vi "Add Data Sharing Framework with UDP Component.vi"(10 "Input System Definition File":path=path "../Assets/Empty.nivssdf", 11 "Output System Definition File":path=path "../Assets/DSF_UDP_Loopback.nivssdf") -> (3 "Created System Definition File":path)   [LabVIEW 2020, in "Data Sharing Framework Scripting Examples.lvlib"]
doc: "Demonstrates using the Data Sharing Framework scripting API to add a UDP plugin for data communication."
uses:
  Data Sharing Framework Scripting Examples.lvlib
  <vilib>/addons/VeriStand Custom Device Scripting APIs/Data Sharing Framework/DSF Core.lvlibp/Typedefs/DSF Engine Framework Configuration.ctl
  <vilib>/addons/VeriStand Custom Device Scripting APIs/Data Sharing Framework/DSF Core.lvlibp/Typedefs/DSF Engine Plugin Configuration.ctl
  <vilib>/addons/VeriStand Custom Device Scripting APIs/Data Sharing Framework/DSF Core.lvlibp/Typedefs/Core Plugin Configuration.ctl
  <vilib>/addons/VeriStand Custom Device Scripting APIs/Data Sharing Framework/DSF Core.lvlibp/Typedefs/DSF Timing Info.ctl
  <vilib>/addons/VeriStand Custom Device Scripting APIs/Data Sharing Framework/DSF Core.lvlibp/Typedefs/DSF Settings Info.ctl
  <vilib>/addons/VeriStand Custom Device Scripting APIs/Data Sharing Framework/DSF Core.lvlibp/Typedefs/DSF Engine Plugin Thread Configuration.ctl
  <vilib>/addons/VeriStand Custom Device Scripting APIs/Data Sharing Framework/DSF Core.lvlibp/Typedefs/Core Thread Configuration.ctl
  <vilib>/addons/VeriStand Custom Device Scripting APIs/Data Sharing Framework/DSF Core.lvlibp/Typedefs/DSF Engine Transfer Group Configuration.ctl
  <vilib>/addons/VeriStand Custom Device Scripting APIs/Data Sharing Framework/DSF Core.lvlibp/Typedefs/Core Group Configuration.ctl
  <vilib>/addons/VeriStand Custom Device Scripting APIs/Data Sharing Framework/DSF Core.lvlibp/Typedefs/DSF Direction.ctl
  <vilib>/addons/VeriStand Custom Device Scripting APIs/Data Sharing Framework/DSF Core.lvlibp/Typedefs/DSF Timeout Behavior.ctl
  <vilib>/addons/VeriStand Custom Device Scripting APIs/Data Sharing Framework/DSF Core.lvlibp/Typedefs/DSF Engine Transfer Configuration.ctl
  <vilib>/addons/VeriStand Custom Device Scripting APIs/Data Sharing Framework/DSF Core.lvlibp/Typedefs/Core Transfer Configuration.ctl
  <vilib>/addons/VeriStand Custom Device Scripting APIs/Data Sharing Framework/DSF Core.lvlibp/Typedefs/DSF Engine Channel Configuration.ctl
  <vilib>/addons/VeriStand Custom Device Scripting APIs/Data Sharing Framework/DSF Core.lvlibp/Typedefs/Core Channel Configuration.ctl
  <vilib>/addons/VeriStand Custom Device Scripting APIs/Data Sharing Framework/DSF Core.lvlibp/Typedefs/DSF Data Type.ctl
  NationalInstruments.VeriStand.SystemDefinitionAPI
  <vilib>/addons/VeriStand Custom Device Scripting APIs/Data Sharing Framework/DSF Core.lvlibp
  <vilib>/addons/VeriStand Custom Device Scripting APIs/Data Sharing Framework/DSF Core.lvlibp/Classes/Configuration/Core/Channel/Channel Configuration.lvclass
  <vilib>/addons/VeriStand Custom Device Scripting APIs/Data Sharing Framework/DSF Core.lvlibp/Classes/Configuration/Core/Transfer/Transfer Configuration.lvclass
  <vilib>/addons/VeriStand Custom Device Scripting APIs/Data Sharing Framework/DSF Core.lvlibp/Classes/Configuration/Core/Group/Group Configuration.lvclass
  <vilib>/addons/VeriStand Custom Device Scripting APIs/Data Sharing Framework/DSF Core.lvlibp/Classes/Configuration/Core/Thread/Thread Configuration.lvclass
  <vilib>/addons/VeriStand Custom Device Scripting APIs/Data Sharing Framework/DSF Core.lvlibp/Classes/Configuration/Core/Plugin/Plugin Configuration.lvclass
  <vilib>/addons/VeriStand Custom Device Scripting APIs/Data Sharing Framework/Data Sharing Framework Custom Device Scripting.lvlib
panel:
  in  "Launch Data Viewer":bool=TRUE
  in  "Data Server Frequency":dbl(ring)=10.0 items=["0.5 Hz"=0.5, "1.0 Hz"=1.0, "2.0 Hz"=2.0, "2.5 Hz"=2.5, "4.0 Hz"=4.0, "5.0 Hz"=5.0, "8.0 Hz"=8.0, "10.0 Hz"=10.0, "12.5 Hz"=12.5, "20.0 Hz"=20.0, "25.0 Hz"=25.0, "40.0 Hz"=40.0, "50.0 Hz"=50.0, "100.0 Hz"=100.0]
  in  "Enable Data Server":bool=TRUE
  in  "Channels":cluster{"Name":string, "Unit":string}[](array[cluster])=[{"Name"="Voltage_an", "Unit"="V"}, {"Name"="Voltage_bn", "Unit"="V"}, {"Name"="Voltage_cn", "Unit"="V"}, {"Name"="Current_a", "Unit"="A"}, {"Name"="Current_b", "Unit"="A"}, {"Name"="Current_c", "Unit"="A"}, {"Name"="Current_n", "Unit"="A"}, {"Name"="Voltage_dc", "Unit"="V"}, {"Name"="Current_dc", "Unit"="A"}, {"Name"="Count", "Unit"="iterations"}]
  # "Overview: Demonstrates using the Data Sharing Framework scripting API to add a UDP plugin for data communication. \n\nInstructions:\n1. Per your application requirements, configure the data channels to share.\n2. Browse to a path to save the system definition file as the output Output System Definition File.  This may be the same as the input file.\n3. Run the VI and verify the resulting system definition file. \n4. Configure addresses and ports in System Explorer."
  # "System Definition Files"
  # "Configure Data Server for Validation"
  # "Data Sharing Framework Channels"
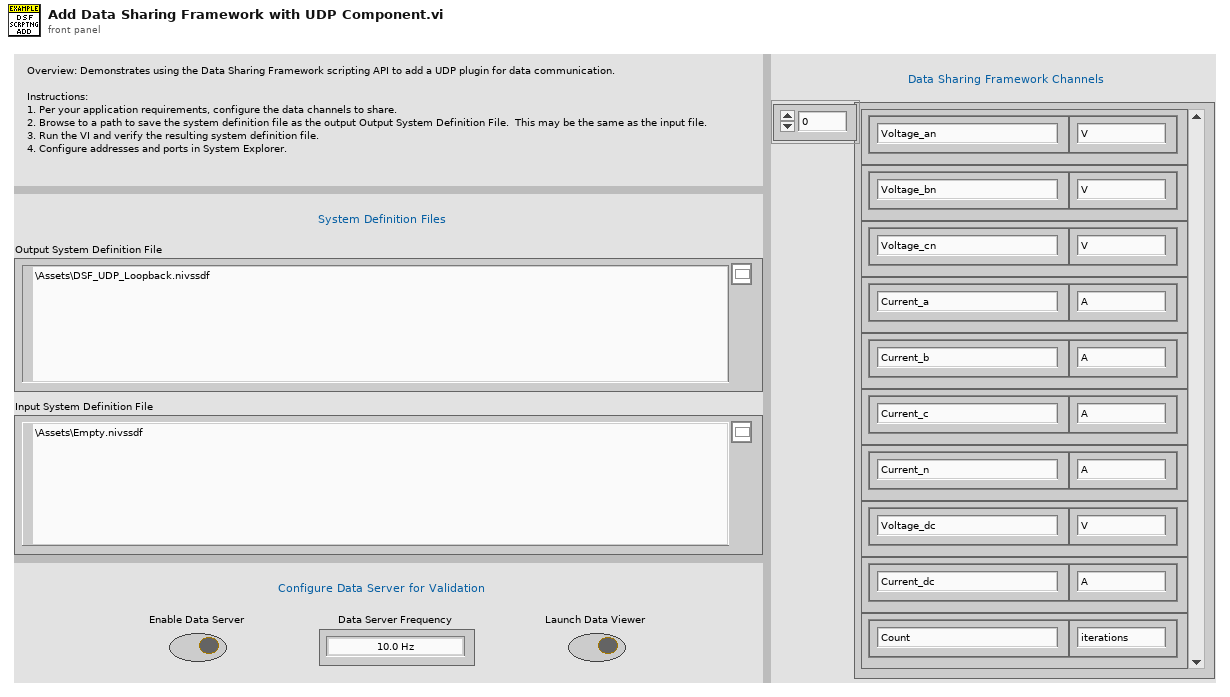
[diagram p1: front panel]
types:
  T1 = typedef "DSF Core.lvlibp/DSF Engine Channel Configuration.ctl" = cluster{"core":T2, "component settings":T4[]}
  T2 = typedef "DSF Core.lvlibp/Channel Configuration.lvclass/Core Channel Configuration.ctl" = cluster{"name":string, "units":string, "engine data type":T3, "string data type":T3, "string offset":u64}
  T3 = typedef "DSF Core.lvlibp/DSF Data Type.ctl" = enum8{"Bool", "SGL", "DBL", "I8", "I16", "I32", "I64", "U8", "U16", "U32", "U64"}
  T4 = typedef "DSF Core.lvlibp/DSF Settings Info.ctl" = cluster{"component":string, "values":cluster{"key":string, "value":string}[]}
  T5 = typedef "DSF Core.lvlibp/DSF Engine Plugin Thread Configuration.ctl" = cluster{"core":T6, "component settings":T4[], "transfer groups":T7[]}
  T6 = typedef "DSF Core.lvlibp/Thread Configuration.lvclass/Core Thread Configuration.ctl" = cluster{"processor":i32, "priority offset":i16}
  T7 = typedef "DSF Core.lvlibp/DSF Engine Transfer Group Configuration.ctl" = cluster{"core":T8, "component settings":T4[], "transfers":T12[]}
  T8 = typedef "DSF Core.lvlibp/Group Configuration.lvclass/Core Group Configuration.ctl" = cluster{"name":string, "direction":T9, "cycle timing":T10, "timeout behavior":T11, "enable conversion":bool}
  T9 = typedef "DSF Core.lvlibp/DSF Direction.ctl" = enum8{"Tx", "Rx"}
  T10 = typedef "DSF Core.lvlibp/DSF Timing Info.ctl" = cluster{"priority":u64, "decimation":u64, "offset":u64}
  T11 = typedef "DSF Core.lvlibp/DSF Timeout Behavior.ctl" = enum8{"Increment Late Count", "Throw Error"}
  T12 = typedef "DSF Core.lvlibp/DSF Engine Transfer Configuration.ctl" = cluster{"core":T13, "component settings":T4[], "channels":T1[]}
  T13 = typedef "DSF Core.lvlibp/Transfer Configuration.lvclass/Core Transfer Configuration.ctl" = cluster{"name":string}
  T14 = typedef "DSF Core.lvlibp/DSF Engine Plugin Configuration.ctl" = cluster{"core":T15, "component settings":T4[], "threads":T5[]}
  T15 = typedef "DSF Core.lvlibp/Plugin Configuration.lvclass/Core Plugin Configuration.ctl" = cluster{"name":string, "components":string[], "cycle timing":T10}
  T16 = typedef "DSF Core.lvlibp/DSF Engine Framework Configuration.ctl" = cluster{"plugins":T14[]}
  T17 = typedef "Custom Device API.lvlib/Custom Device Item Ref.ctl" = u64
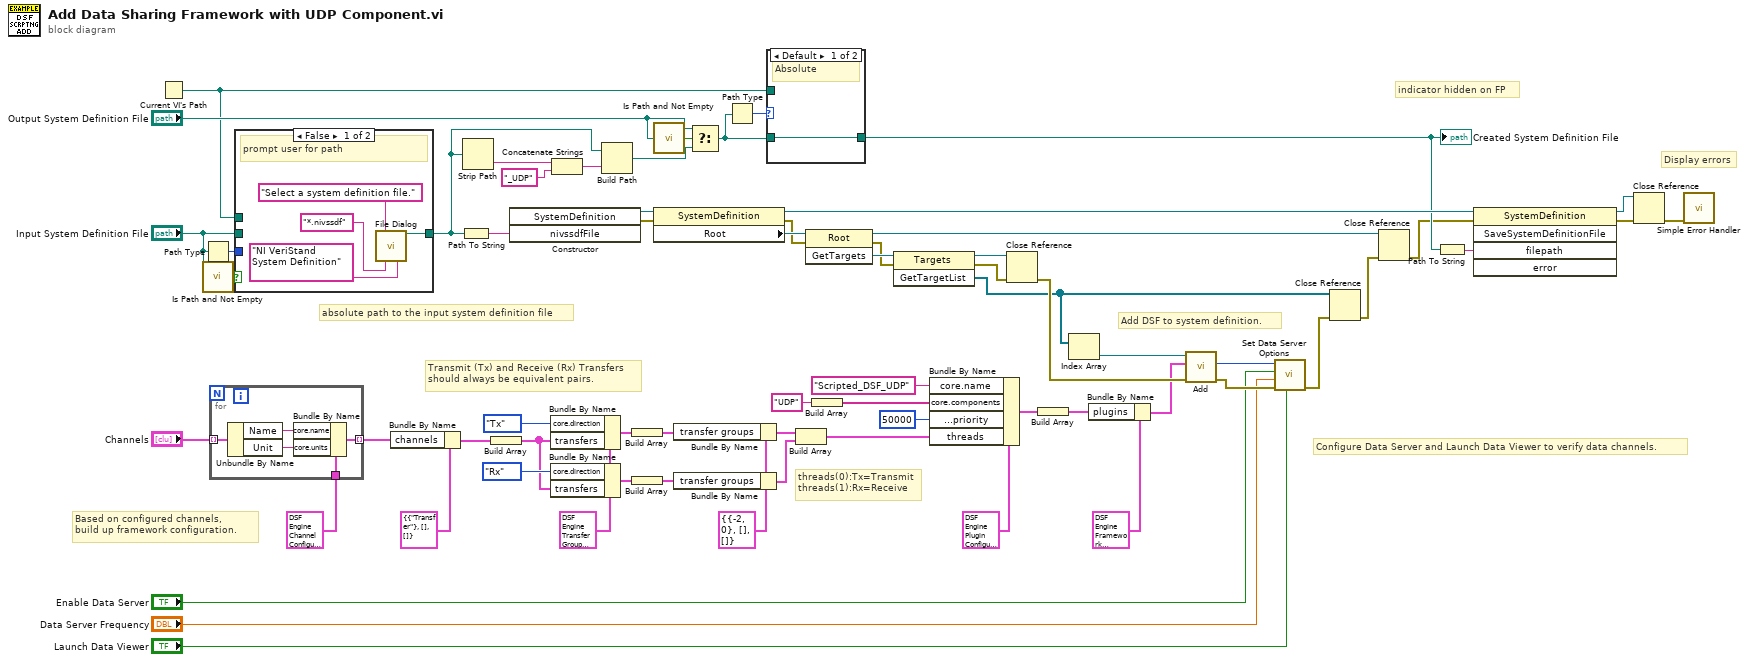
[diagram p0: block diagram]
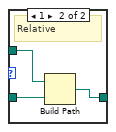
[diagram p2: hidden frame]
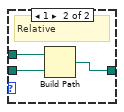
[diagram p4: hidden frame]
diagram:
  w21 = T5 {"core"={"processor"=-2, "priority offset"=0}, "component settings"=[], "transfer groups"=[]} ("element")
  w28 = T7 {"core"={"name"="Group", "direction"=enum."Tx", "cycle timing"={"priority"=100, "decimation"=1, "offset"=0}, "timeout behavior"=enum."Increment Late Count", "enable conversion"=FALSE}, "component settings"=[], "transfers"=[]} ("element")
  # "indicator hidden on FP"
  # "Transmit (Tx) and Receive (Rx) Transfers \nshould always be equivalent pairs."
  # "absolute path to the input system definition file"
  # "Display errors"
  # "Add DSF to system definition."
  # "threads(0):Tx=Transmit\nthreads(1):Rx=Receive"
  # "Based on configured channels, \nbuild up framework configuration."
  # "Configure Data Server and Launch Data Viewer to verify data channels."
  n1 = Current VI's Path() -> (path=w2:path)
  n2 = Path Type(1:"Input System Definition File") -> (0:w66:i16)
  n3 = call <vilib>:"Is Path and Not Empty.vi"("path"="Input System Definition File") -> ("Is Path and Not Empty?"=w64:bool)  [unwired: 4 in]
  n4 = for {
    tunnel: "Channels" -> [w71] mode=indexing
    tunnel: [w68] -> w32 mode=indexing
    tunnel: T1 {"core"={"name"="Voltage", "units"="V", "engine data type"=enum."DBL", "string data type"=enum."DBL", "string offset"=0}, "component settings"=[]} ("channel configuration") -> [w67]
    n5 = Unbundle By Name(w71) -> ("Name"=w70:string, "Unit"=w69:string)
    n6 = Bundle By Name(cluster=w67, "core.name"=w70, "core.units"=w69) -> (w68:T1)
  }
  n7 = case shown="False" w64 {
    tunnel: w66 -> [_ w79]
    tunnel: "Input System Definition File" -> [_ w78]
    tunnel: [w72 w77] -> w9
    tunnel: w2 -> [_ w76]
    frame False {
      # "prompt user for path"
      n8 = call "File Dialog"("prompt"="Select a system definition file.", "pattern (all files)"="*.nivssdf", "pattern label"="NI VeriStand System Definition") -> ("selected path"=w72:path)  [unwired: 9 in, 3 out]
    }
    frame True {
      # "input path converted to absolute"
      n9 = case shown="Default" w79 {
        tunnel: w76 -> [_ w83]
        tunnel: w78 -> [w80 w82]
        tunnel: [w80 w81] -> w77
        frame Default {
          # "Absolute"
        }
        frame 1 {
          # "Relative"
          n10 = Build Path(base path=w83, name or relative path=w82) -> (appended path=w81:path)
        }
      }
    }
  }
  n11 = Bundle By Name(cluster=T12 {"core"={"name"="Transfer"}, "component settings"=[], "channels"=[]} ("output cluster"), "channels"=w32) -> (w30:T12)
  n12 = Path To String(path=w9) -> (string=w55:string)
  n13 = Strip Path(path=w9) -> (name=w52:string)  [unwired: 1 out]
  n14 = Build Array(w30) -> (w29:T12[])
  n15 = constructor class="SystemDefinition"("nivssdfFile"=w55) -> (reference out=w57:refnum<k24>, error out=w56:errorcluster)  [unwired: 3 in, 2 out]
  n16 = Bundle By Name(cluster=w28, "core.direction"=DSF_Direction."Tx", "transfers"=w29) -> (w27:T7)
  n17 = Bundle By Name(cluster=w28, "core.direction"=DSF_Direction."Rx", "transfers"=w29) -> (w26:T7)
  n18 = Concatenate Strings(w52, "_UDP" ("string")) -> (w50:string)
  n19 = Build Path(base path=w9, name or relative path=w50) -> (appended path=w4:path)
  n20 = Build Array(w27) -> (w24:T7[])
  n21 = Build Array(w26) -> (w25:T7[])
  n22 = call <vilib>:"Is Path and Not Empty.vi"("path"="Output System Definition File") -> ("Is Path and Not Empty?"=w53:bool)  [unwired: 4 in]
  n23 = property class="SystemDefinition"(reference=w57, error in=w56) -> (reference out=w45:refnum<k24>, error out=w58:errorcluster, "Root"=w59:refnum<k24>)
  n24 = Bundle By Name(cluster=w21, "transfer groups"=w24) -> (w23:T5)
  n25 = Bundle By Name(cluster=w21, "transfer groups"=w25) -> (w22:T5)
  n26 = Select(t="Output System Definition File", s=w53, f=w4) -> (s? t:f=w49:path)
  n27 = Path Type(1:w49) -> (0:w54:i16)
  n28 = case shown="Default" w54 {
    tunnel: w2 -> [_ w87]
    tunnel: w49 -> [w84 w86]
    tunnel: [w84 w85] -> w41
    frame Default {
      # "Absolute"
    }
    frame 1 {
      # "Relative"
      n29 = Build Path(base path=w87, name or relative path=w86) -> (appended path=w85:path)
    }
  }
  "Created System Definition File" <- w41
  n30 = Build Array(w23, w22) -> (w20:T5[])
  n31 = invoke class="Root" method="GetTargets"(reference=w59, error in=w58) -> (reference out=w47:refnum<k24>, error out=w60:errorcluster, "GetTargets"=w61:refnum<k24>)  [unwired: 1 in]
  n32 = Build Array("UDP" ("class")) -> (w37:string[])
  n33 = invoke class="Targets" method="GetTargetList"(reference=w61, error in=w60) -> (reference out=w63:refnum<k24>, error out=w62:errorcluster, "GetTargetList"=w1:refnum<k24>[])  [unwired: 1 in]
  n34 = Bundle By Name(cluster=T14 {"core"={"name"="", "components"=["UDP"], "cycle timing"={"priority"=10000, "decimation"=1, "offset"=0}}, "component settings"=[], "threads"=[{"core"={"processor"=-2, "priority offset"=0}, "component settings"=[], "transfer groups"=[{"core"={"name"="Group", "direction"=enum."Tx", "cycle timing"={"priority"=100, "decimation"=1, "offset"=0}, "timeout behavior"=enum."Increment Late Count", "enable conversion"=FALSE}, "component settings"=[], "transfers"=[{"core"={"name"="Transfer"}, "component settings"=[], "channels"=[{"core"={"name"="Voltage", "units"="V", "engine data type"=enum."DBL", "string data type"=enum."DBL", "string offset"=0}, "component settings"=[]}, {"core"={"name"="Current", "units"="A", "engine data type"=enum."DBL", "string data type"=enum."DBL", "string offset"=0}, "component settings"=[]}]}]}]}, {"core"={"processor"=-2, "priority offset"=0}, "component settings"=[], "transfer groups"=[{"core"={"name"="Group", "direction"=enum."Rx", "cycle timing"={"priority"=100, "decimation"=1, "offset"=0}, "timeout behavior"=enum."Increment Late Count", "enable conversion"=FALSE}, "component settings"=[], "transfers"=[{"core"={"name"="Transfer"}, "component settings"=[], "channels"=[{"core"={"name"="Voltage", "units"="V", "engine data type"=enum."DBL", "string data type"=enum."DBL", "string offset"=0}, "component settings"=[]}, {"core"={"name"="Current", "units"="A", "engine data type"=enum."DBL", "string data type"=enum."DBL", "string offset"=0}, "component settings"=[]}]}]}]}]} ("Plugin Configuration"), "core.name"="Scripted_DSF_UDP", "core.components"=w37, "core.cycle timing.priority"=u64 50000, "threads"=w20) -> (w19:T14)
  n35 = Close Reference(reference=w63, error in (no error)=w62) -> (error out=w11:errorcluster)
  n36 = Build Array(w19) -> (w17:T14[])
  n37 = Index Array(array=w1) -> (element=w13:refnum<k24>)  [unwired: 1 in]
  n38 = Bundle By Name(cluster=T16 {"plugins"=[{"core"={"name"="", "components"=["UDP"], "cycle timing"={"priority"=10000, "decimation"=1, "offset"=0}}, "component settings"=[], "threads"=[{"core"={"processor"=-2, "priority offset"=0}, "component settings"=[], "transfer groups"=[{"core"={"name"="Group", "direction"=enum."Tx", "cycle timing"={"priority"=100, "decimation"=1, "offset"=0}, "timeout behavior"=enum."Increment Late Count", "enable conversion"=FALSE}, "component settings"=[], "transfers"=[{"core"={"name"="Transfer"}, "component settings"=[], "channels"=[{"core"={"name"="Voltage", "units"="V", "engine data type"=enum."DBL", "string data type"=enum."DBL", "string offset"=0}, "component settings"=[]}, {"core"={"name"="Current", "units"="A", "engine data type"=enum."DBL", "string data type"=enum."DBL", "string offset"=0}, "component settings"=[]}]}]}]}, {"core"={"processor"=-2, "priority offset"=0}, "component settings"=[], "transfer groups"=[{"core"={"name"="Group", "direction"=enum."Rx", "cycle timing"={"priority"=100, "decimation"=1, "offset"=0}, "timeout behavior"=enum."Increment Late Count", "enable conversion"=FALSE}, "component settings"=[], "transfers"=[{"core"={"name"="Transfer"}, "component settings"=[], "channels"=[{"core"={"name"="Voltage", "units"="V", "engine data type"=enum."DBL", "string data type"=enum."DBL", "string offset"=0}, "component settings"=[]}, {"core"={"name"="Current", "units"="A", "engine data type"=enum."DBL", "string data type"=enum."DBL", "string offset"=0}, "component settings"=[]}]}]}]}]}]} ("framework configuration"), "plugins"=w17) -> (w8:T16)
  n39 = call <vilib>:"Add.vi"("error in"=w11, "framework configuration"=w8, "target in"=w13) -> ("error out"=w12:errorcluster, "data sharing framework custom device"=w14:T17)  [unwired: 6 in, 1 out]
  n40 = call <vilib>:"Set Data Server Options.vi"("launch data viewer"="Launch Data Viewer", "error in"=w12, "data server frequency (Hz)"="Data Server Frequency", "enable data server"="Enable Data Server", "data sharing framework custom device in"=w14) -> ("error out"=w10:errorcluster)  [unwired: 4 in, 2 out]
  n41 = Close Reference(reference=w1, error in (no error)=w10) -> (error out=w48:errorcluster)
  n42 = Close Reference(reference=w47, error in (no error)=w48) -> (error out=w40:errorcluster)
  n43 = Path To String(path=w41) -> (string=w46:string)
  n44 = invoke class="SystemDefinition" method="SaveSystemDefinitionFile"(reference=w45, error in=w40, "filepath"=w46) -> (reference out=w43:refnum<k24>, error out=w44:errorcluster)  [unwired: 2 in, 3 out]
  n45 = Close Reference(reference=w43, error in (no error)=w44) -> (error out=w42:errorcluster)
  n46 = call <vilib>:"Simple Error Handler.vi"("error in (no error)"=w42) -> ()  [unwired: 1 in, 8 out]
